vi "UpdateMatlabParamDataToVartiant.vi"(0 "Type (or value to update)":variant, 1 "MatlabDataBundle":T1, 2 "NamePath":string[](array[string]), 3 "Namepath Index":i32, 5 "Info collection refrence in":refnum<vi>, 6 "Allow Variant Values (f)":bool, 18 "Info":string[](array[string])) -> (14 "Value":variant, 19 "Info collection refrence out":refnum<vi>)   [LabVIEW 2017]
uses:
  Types/MatlabDataBundle.ctl
  Types/MatlabDataType.ctl
panel:
  out "Updating index":i32
  out "Updating Name":string
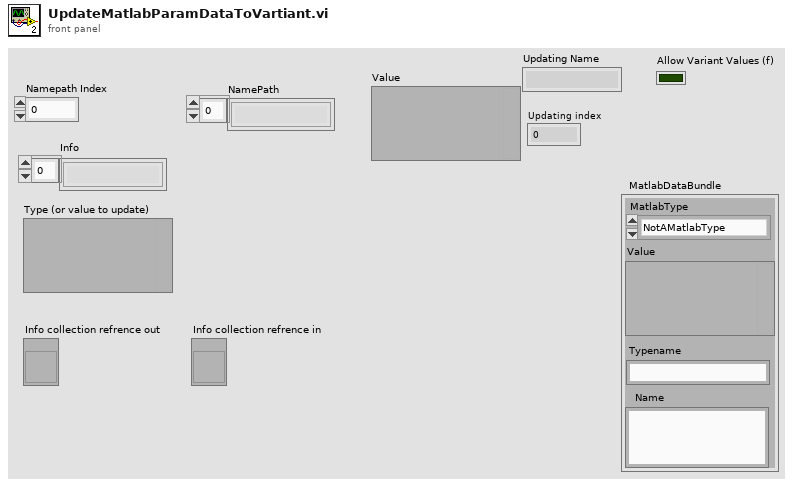
[diagram p1: front panel]
types:
  T1 = typedef "MatlabDataBundle.ctl" = cluster{"MatlabType":T2, "Value":variant, "Name":string, "Typename":string}
  T2 = typedef "MatlabDataType.ctl" = enum16{"NotAMatlabType", "Real", "Complex", "String", "Boolean"}
  T3 = typedef "NI_Data Type.lvlib/Data Type.ctl" = enum8{"Invalid Type", "Void", "I8", "I16", "I32", "I64", "U8", "U16", "U32", "U64", "Single Float", "Double Float", "Extended Float", "Single Complex", "Double Complex", "Extended Complex", "Enum U8", "Enum U16", "Enum U32", "Enum U64", "Single Float With Unit", "Double Float With Unit", "Extended Float With Unit", "Single Complex with Unit", "Double Complex with Unit", "Extended Complex with Unit", "Boolean", "String", "Path", "Picture", "Tag", "Array", "Cluster", "Variant", "LV Variant", "Waveform", "Timestamp", "Digital Waveform", "Digital Data", "ExpressData", "Refnum", "External Data", "VI", "Poly VI", "LabVIEW Class Instance", "Fixed Point"}
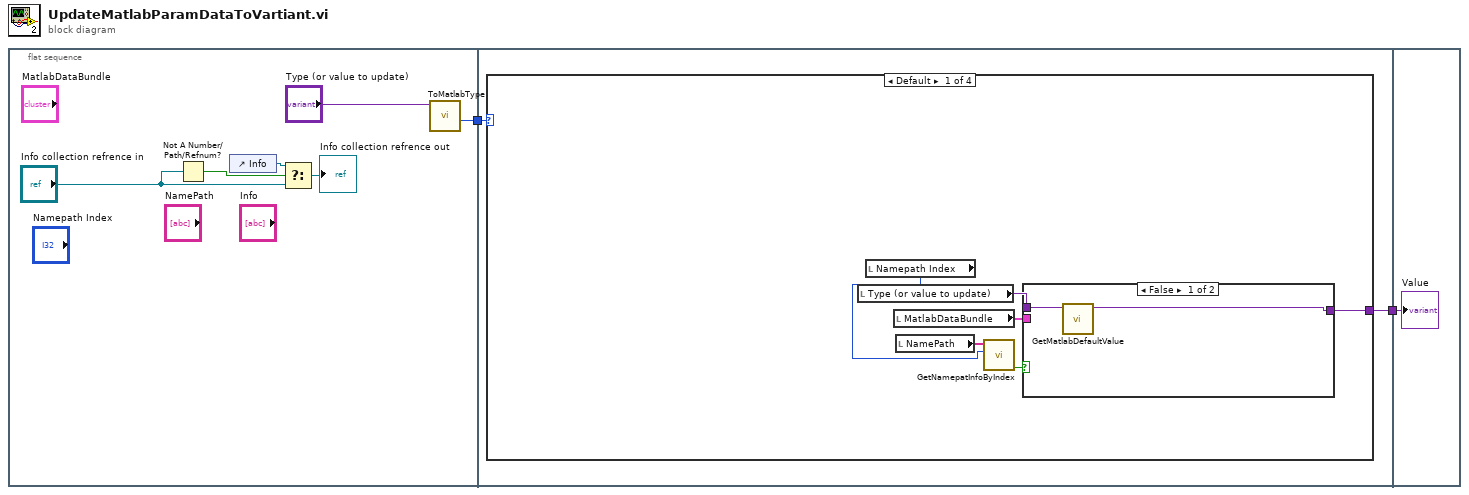
[diagram p0: block diagram]
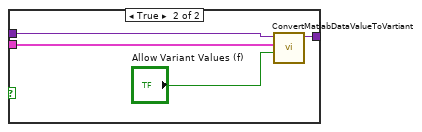
[diagram p2: hidden frame]
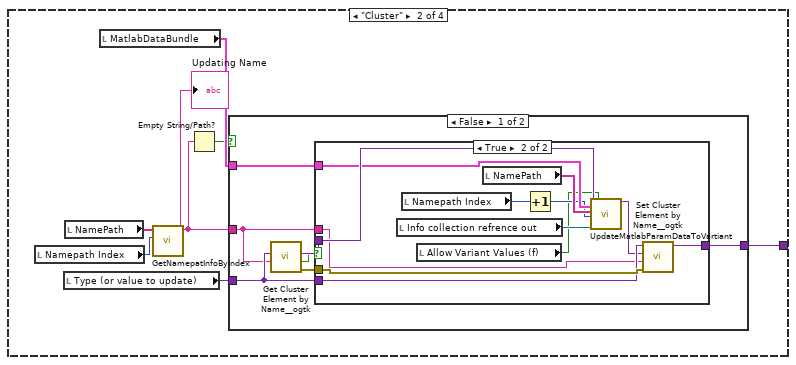
[diagram p3: hidden frame]
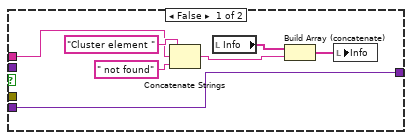
[diagram p4: hidden frame]
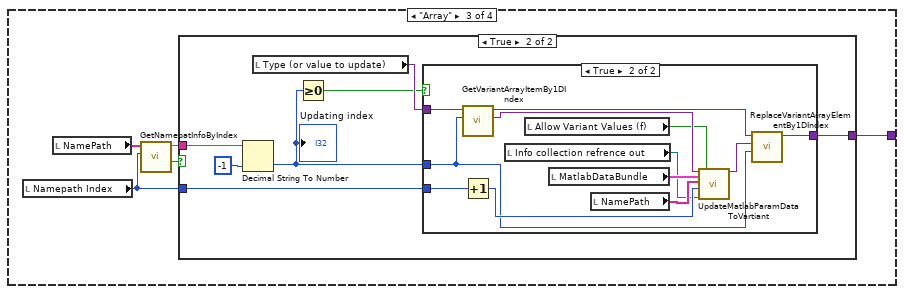
[diagram p6: hidden frame]
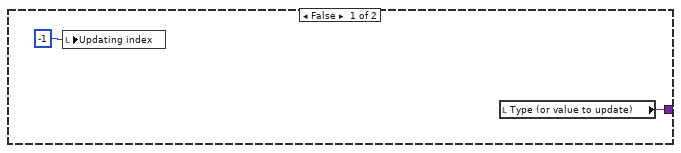
[diagram p7: hidden frame]
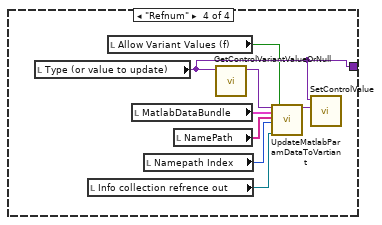
[diagram p9: hidden frame]
diagram:
  n1 = flat-sequence {
    tunnel: [w7] -> w2
    tunnel: w2 -> [w9]
    tunnel: [w10] -> w1
    tunnel: w1 -> [w92]
    frame #0 {
      n2 = Not A Number/Path/Refnum?(number/path/refnum="Info collection refrence in") -> (NaN/Path/Refnum?=w6:bool)
      n3 = control-ref of="Info"() -> (w5:refnum<vi>)
      n4 = Select(t=w5, s=w6, f="Info collection refrence in") -> (s? t:f=→"Info collection refrence out":refnum<vi>)
      n5 = call "ToMatlabType.vi"("Value"="Type (or value to update)") -> ("Type"=w7:T3)  [unwired: 6 in, 4 out]
    }
    frame #1 {
      n6 = case shown="Default" w9 {
        tunnel: [w16 w27 w61 w89] -> w10
        frame Default {
          n7 = local read "Type (or value to update)"() -> (w15:variant)
          n8 = local read "Namepath Index"() -> (w13:i32)
          n9 = local read "MatlabDataBundle"() -> (w14:T1)
          n10 = local read "NamePath"() -> (w12:string[])
          n11 = call "GetNamepatInfoByIndex.vi"("Namepath Index"=w13, "NamePath"=w12) -> ("At array end"=w11:bool)  [unwired: 7 in, 2 out]
          n12 = case shown="False" w11 {
            tunnel: [w18 w22] -> w16
            tunnel: w15 -> [w17 w21]
            tunnel: w14 -> [_ w20]
            frame False {
              n13 = call "GetMatlabDefaultValue.vi"("From Value Type"=w17) -> ("Default Value"=w18:variant)  [unwired: 10 in]
            }
            frame True {
              n14 = call "ConvertMatlabDataValueToVartiant.vi"("Allow Variant Values (f)"="Allow Variant Values (f)", "MatlabDataBundle"=w20, "Data Value"=w21) -> ("Value"=w22:variant)  [unwired: 8 in]
            }
          }
        }
        frame "Cluster" {
          n15 = local read "Namepath Index"() -> (w23:i32)
          n16 = local read "Type (or value to update)"() -> (w28:variant)
          n17 = local read "NamePath"() -> (w25:string[])
          n18 = local read "MatlabDataBundle"() -> (w29:T1)
          n19 = call "GetNamepatInfoByIndex.vi"("Namepath Index"=w23, "NamePath"=w25) -> ("Name"=w24:string)  [unwired: 7 in, 2 out]
          "Updating Name" <- w24
          n20 = Empty String/Path?(string/path=w24) -> (empty?=w26:bool)
          n21 = case shown="False" w26 {
            tunnel: w29 -> [w35 _]
            tunnel: w28 -> [w33 w56]
            tunnel: [w32 w56] -> w27
            tunnel: w24 -> [w31 _]
            frame False {
              n22 = call <userlib>:"Get Cluster Element by Name__ogtk.vi"("Element Name"=w31, "Cluster"=w33) -> ("error out"=w34:errorcluster, "found?"=w30:bool, "VElement"=w36:variant)  [unwired: 7 in]
              n23 = case shown="True" w30 {
                tunnel: w36 -> [_ w55]
                tunnel: w35 -> [_ w54]
                tunnel: w34 -> [_ w53]
                tunnel: w33 -> [w43 w52]
                tunnel: [w43 w51] -> w32
                tunnel: w31 -> [w39 w49]
                frame False {
                  n24 = Concatenate Strings("Cluster element ", w39, " not found") -> (w41:string)
                  n25 = local read "Info"() -> (w42:string[])
                  n26 = Build Array (concatenate)(w42, w41) -> (w37:string[])
                  n27 = local write "Info"(w37) -> ()
                }
                frame True {
                  n28 = local read "Info collection refrence out"() -> (w48:refnum<vi>)
                  n29 = local read "Namepath Index"() -> (w46:i32)
                  n30 = local read "Allow Variant Values (f)"() -> (w44:bool)
                  n31 = local read "NamePath"() -> (w47:string[])
                  n32 = Increment(x=w46) -> (x+1=w45:i32)
                  n33 = call "UpdateMatlabParamDataToVartiant.vi"("Type (or value to update)"=w55, "MatlabDataBundle"=w54, "NamePath"=w47, "Namepath Index"=w45, "Info collection refrence in"=w48, "Allow Variant Values (f)"=w44) -> ("Value"=w50:variant)  [unwired: 12 in, 1 out]
                  n34 = call <userlib>:"Set Cluster Element by Name__ogtk.vi"("error in (no error)"=w53, "Element Name (\"\": New Element Data Name)"=w49, "New Element Value"=w50, "Cluster"=w52) -> ("VCluster out"=w51:variant)  [unwired: 5 in, 2 out]
                }
              }
            }
            frame True {
            }
          }
        }
        frame "Array" {
          n35 = local read "Namepath Index"() -> (w60:i32)
          n36 = local read "NamePath"() -> (w59:string[])
          n37 = call "GetNamepatInfoByIndex.vi"("Namepath Index"=w60, "NamePath"=w59) -> ("Namepart found?"=w57:bool, "Name"=w58:string)  [unwired: 7 in, 1 out]
          n38 = case shown="True" w57 {
            tunnel: [w63 w69] -> w61
            tunnel: w60 -> [_ w65]
            tunnel: w58 -> [_ w64]
            frame False {
              n39 = local write "Updating index"(-1 ("Updating index")) -> ()
              n40 = local read "Type (or value to update)"() -> (w63:variant)
            }
            frame True {
              n41 = Decimal String To Number(string=w64, default (0L)=-1 ("default (0 I32)")) -> (number=w67:i32)  [unwired: 1 in, 1 out]
              "Updating index" <- w67
              n42 = local read "Type (or value to update)"() -> (w70:variant)
              n43 = Greater Or Equal To 0?(x=w67) -> (x >= 0?=w66:bool)
              n44 = case shown="True" w66 {
                tunnel: w70 -> [w71 w83]
                tunnel: w67 -> [_ w73]
                tunnel: [w71 w77] -> w69
                tunnel: w65 -> [_ w76]
                frame False {
                }
                frame True {
                  n45 = call "GetVariantArrayItemBy1DIndex.vi"("Index"=w73, "Array in"=w83) -> ("Array Element"=w80:variant, "Array out"=w78:variant)  [unwired: 8 in]
                  n46 = Increment(x=w76) -> (x+1=w75:i32)
                  n47 = local read "Info collection refrence out"() -> (w74:refnum<vi>)
                  n48 = local read "Allow Variant Values (f)"() -> (w72:bool)
                  n49 = local read "MatlabDataBundle"() -> (w81:T1)
                  n50 = local read "NamePath"() -> (w82:string[])
                  n51 = call "UpdateMatlabParamDataToVartiant.vi"("Type (or value to update)"=w80, "MatlabDataBundle"=w81, "NamePath"=w82, "Namepath Index"=w75, "Info collection refrence in"=w74, "Allow Variant Values (f)"=w72) -> ("Value"=w79:variant)  [unwired: 12 in, 1 out]
                  n52 = call "ReplaceVariantArrayElementBy1DIndex.vi"("Index (1D)"=w73, "Value"=w79, "Array in"=w78) -> ("Array out"=w77:variant)  [unwired: 8 in]
                }
              }
            }
          }
        }
        frame "Refnum" {
          n53 = local read "Type (or value to update)"() -> (w89:variant)
          n54 = local read "Info collection refrence out"() -> (w88:refnum<vi>)
          n55 = local read "Allow Variant Values (f)"() -> (w84:bool)
          n56 = local read "MatlabDataBundle"() -> (w87:T1)
          n57 = local read "Namepath Index"() -> (w85:i32)
          n58 = local read "NamePath"() -> (w86:string[])
          n59 = call "GetControlVariantValueOrNull.vi"("ControlVariant"=w89) -> ("Value"=w91:variant)  [unwired: 9 in, 1 out]
          n60 = call "UpdateMatlabParamDataToVartiant.vi"("Type (or value to update)"=w91, "MatlabDataBundle"=w87, "NamePath"=w86, "Namepath Index"=w85, "Info collection refrence in"=w88, "Allow Variant Values (f)"=w84) -> ("Value"=w90:variant)  [unwired: 12 in, 1 out]
          n61 = call "SetControlValue.vi"("Value"=w90, "ControlVariant"=w89) -> ()  [unwired: 9 in, 1 out]
        }
      }
    }
    frame #2 {
      "Value" <- w92
    }
  }
